vi "CloseSink.vi"(8 "error in (no error)":errorcluster, 11 "ConsoleAppender in":refnum<class "ConsoleAppender.lvclass">) -> (0 "error out":errorcluster, 3 "ConsoleAppender out":refnum<class "ConsoleAppender.lvclass">)   [LabVIEW 2026, in "Lumberjack.lvlib" / "ConsoleAppender.lvclass"]
doc: "No-op: the console has no resource to flush or close. Override of the abstract CloseSink."
uses:
  ConsoleAppender.lvclass
  Appender.lvclass/Appender.lvclass
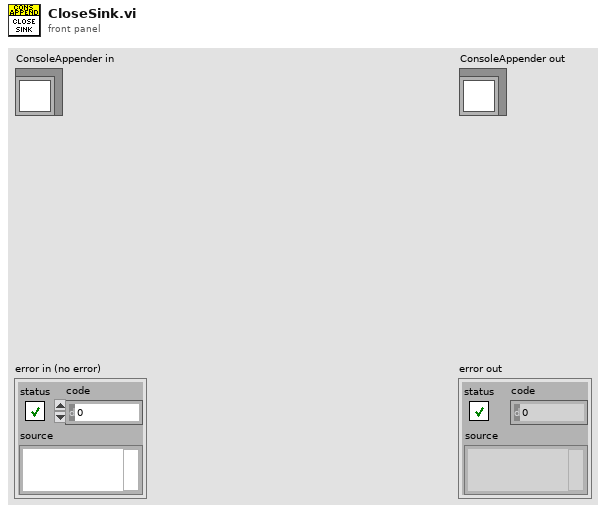
[diagram p1: front panel]
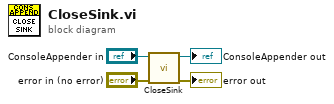
[diagram p0: block diagram]
diagram:
  n1 = call-parent "CloseSink.vi"("error in (no error)"="error in (no error)", "Appender in"="ConsoleAppender in") -> ("error out"=→"error out":errorcluster, "Appender out"=→"ConsoleAppender out":refnum<class "ConsoleAppender.lvclass">)  [unwired: 8 in]
